vi "New_ParseTree_Node.vi"(0 "Parse Tree in":T2[](array[typedef]), 5 "parent":u32, 7 "children":u32[](array[numeric]), 9 "token":string, 11 "NodeType":T1, 12 "line":u32, 13 "position":u32, 14 "display":bool) -> (4 "Parse Tree out":T2[](array[typedef]), 8 "new node index":i32)   [LabVIEW 2021]
uses:
  <resource>/MathScriptParser/Statement.ctl
  <resource>/MathScriptParser/NodeType.ctl
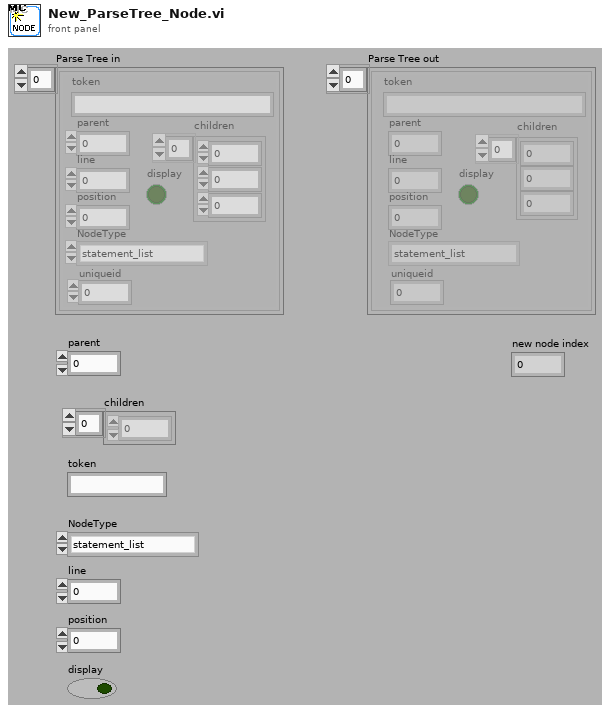
[diagram p1: front panel]
types:
  T1 = typedef "NodeType.ctl" = enum16{"statement_list", "expression_list", "matrix", "row", "command", "function_1_1", "function_1_N", "function_N_1", "function_N_N", "operator", "assignment", "for", "if", "switch", "while", "try", "range", "identifier", "struct_field", "constant", "udfunction_1_1", "udfunction_1_N", "udfunction_N_1", "udfunction_N_N", "udfunction_0_0", "udfunction_0_1", "udfunction_0_N", "udfunction_1_0", "udfunction_N_0", "function_0_1", "function_0_N", "struct_ref", "array_ref", "cell_array_ref", "cell_matrix"}
  T2 = typedef "Statement.ctl" = cluster{"parent":u32, "children":u32[], "token":string, "NodeType":T1, "line":u32, "display":bool, "position":u32, "uniqueid":u32}
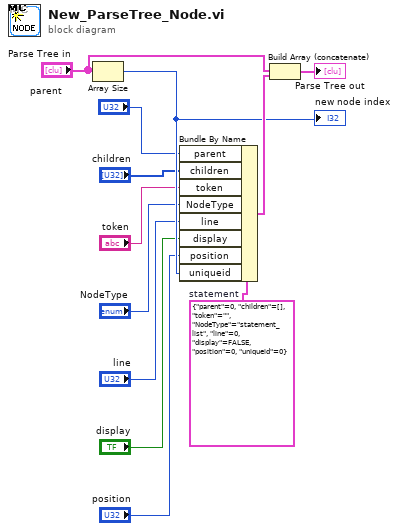
[diagram p0: block diagram]
diagram:
  w1 = T2 {"parent"=0, "children"=[], "token"="", "NodeType"=enum."statement_list", "line"=0, "display"=FALSE, "position"=0, "uniqueid"=0}  # statement
  n1 = Array Size(array="Parse Tree in") -> (size(s)=w9:i32)
  "new node index" <- w9
  n2 = Bundle By Name(cluster=w1, "parent"="parent", "children"="children", "token"="token", "NodeType"="NodeType", "line"="line", "display"="display", "position"="position", "uniqueid"=w9) -> (w10:T2)
  n3 = Build Array (concatenate)("Parse Tree in", w10) -> (→"Parse Tree out":T2[])
